vi "AV Write Single.vi"(8 "error in":errorcluster, 9 "Channel Index":i32=1, 10 "Humidity AV":dbl, 11 "Pressure Actual Value in":refnum<class "Pressure Actual Value.lvclass">) -> (0 "error out":errorcluster, 3 "Pressure Actual Value out":refnum<class "Pressure Actual Value.lvclass">)   [LabVIEW 2023, in "Pressure Actual Value.lvclass"]
uses:
  Pressure Actual Value.lvclass
  Parents/Actual Value/Actual Value.lvclass
  Pressure Actual Value.lvclass/Pressure Actual Value.ctl
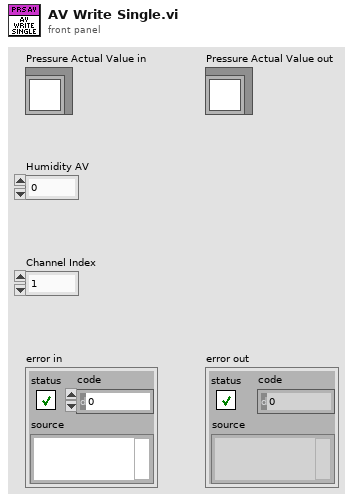
[diagram p1: front panel]
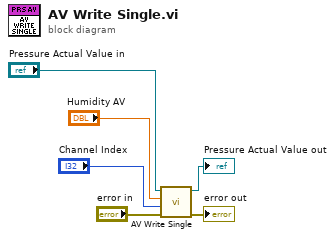
[diagram p0: block diagram]
diagram:
  n1 = call-parent "AV Write Single.vi"("error in"="error in", "Channel Index"="Channel Index", "Actual Value"="Humidity AV", "Actual Value in"="Pressure Actual Value in") -> ("error out"=→"error out":errorcluster, "Actual Value out"=→"Pressure Actual Value out":refnum<class "Pressure Actual Value.lvclass">)  [unwired: 6 in]
